vi "RPN From This Terminal.vi"(11 "output ref":refnum<vi>) -> (3 "Array":T1[](array[typedef]))   [LabVIEW 2018, in "RPN.lvlib"]
uses:
  RPN.lvlib
  Node Type Def.ctl
panel:
  out "error out":errorcluster
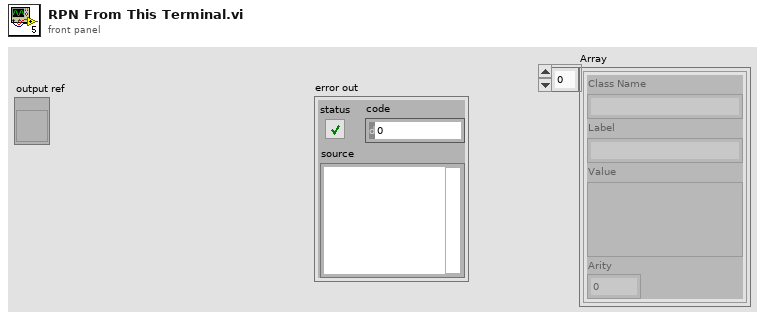
[diagram p1: front panel]
types:
  T1 = typedef "RPN.lvlib/Node Type Def.ctl" = cluster{"Class Name":string, "Label":string, "Value":variant, "Arity":u8}
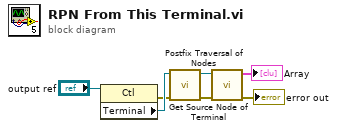
[diagram p0: block diagram]
diagram:
  n1 = property class="Ctl"(reference="output ref") -> (error out=w5:errorcluster, "Terminal"=w6:refnum<vi>)  [unwired: 1 in, 1 out]
  n2 = call "Get Source Node of Terminal.vi"("error in (no error)"=w5, "Terminal in"=w6) -> ("error out"=w3:errorcluster, "Generic out"=w4:refnum<vi>)  [unwired: 8 in]
  n3 = call "Postfix Traversal of Nodes.vi"("error in (no error)"=w3, "Generic in"=w4) -> ("error out"=→"error out":errorcluster, "Array"=→"Array":T1[])  [unwired: 8 in]
